vi "SavePics1.vi"(2 "error IN":errorcluster, 3 "default name":string="Proces_Img", 4 "Image Dst IN":T1) -> (0 "error out":errorcluster)   [LabVIEW 2017]
doc: "Saving of pictures in *png format using the file dialog"
uses:
  <vilib>/vision/Image Controls.llb/IMAQ Image.ctl
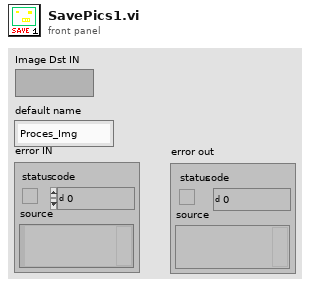
[diagram p1: front panel]
types:
  T1 = typedef "IMAQ Image.ctl" = refnum<image>
  T2 = typedef "Image Type" = u32
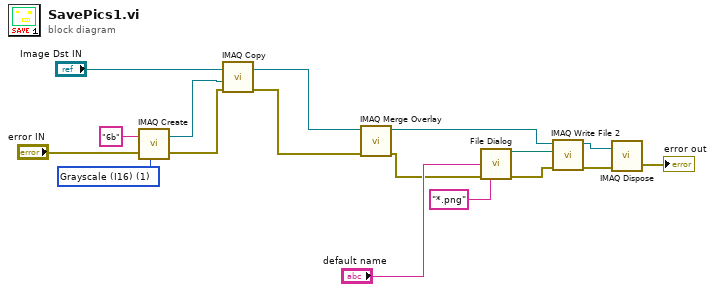
[diagram p0: block diagram]
diagram:
  w7 = T2 1 items=["Grayscale (U8)", "Grayscale (I16)", "Grayscale (SGL)", "Complex (CSG)", "RGB (U32)", "HSL (U32)", "RGB (U64)", "Grayscale (U16)"] ("Image Type")
  n1 = call "IMAQ Create"("Image Name"="6b", "Image Type"=w7, "error in (no error)"="error IN") -> ("New Image"=w4:T1, "error out"=w3:errorcluster)  [unwired: 2 in]
  n2 = call "IMAQ Copy"("error in (no error)"=w3, "Image Dst"=w4, "Image Src"="Image Dst IN") -> ("error out"=w2:errorcluster, "Image Dst Out"=w1:T1)  [unwired: 3 in]
  n3 = call "IMAQ Merge Overlay"("error in (no error)"=w2, "Image Src"=w1) -> ("error out"=w9:errorcluster, "Image Dst Out"=w8:T1)  [unwired: 8 in]
  n4 = call "File Dialog"("default name"="default name", "error in"=w9, "pattern (all files)"="*.png") -> ("selected path"=w13:path, "error out"=w15:errorcluster)  [unwired: 9 in, 2 out]
  n5 = call-poly "IMAQ Write File 2"("error in (no error)"=w15, "File Path"=w13, "Image"=w8) -> ("error out"=w16:errorcluster, "Image Out (duplicate)"=w17:T1)  [unwired: 7 in]
  n6 = call "IMAQ Dispose"("Image"=w17, "error in (no error)"=w16) -> ("error out"=→"error out":errorcluster)  [unwired: 4 in]
